vi "TwReadRawData.vi"(3 "error in (no error)":errorcluster, 4 "buffer":u8[](array[numeric]), 5 "filename":string, 6 "bufferSize in":i32, 7 "writeIndex":i32, 8 "bufIndex":i32, 9 "channel":i32) -> (0 "buffer out":u8[](array[numeric]), 1 "bufferSize out":i32, 2 "error out":errorcluster)   [LabVIEW 2009]
uses:
  TwH5Dll.dll
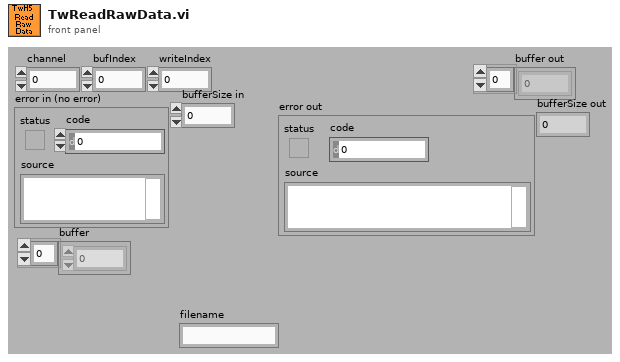
[diagram p1: front panel]
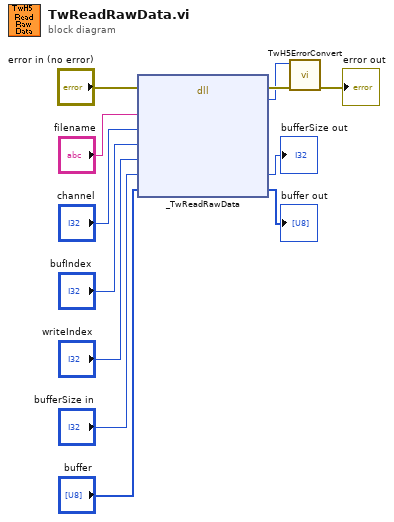
[diagram p0: block diagram]
diagram:
  n1 = dll-call lib="C:/src/85_TofDaq_current/DllWrappers/LabView/TwH5Dll/TwH5Dll.dll" fn="_TwReadRawData"(error in="error in (no error)", "filename"="filename", "channel"="channel", "bufIndex"="bufIndex", "writeIndex"="writeIndex", "bufferSize"="bufferSize in", "buffer"="buffer") -> (error out=w11:errorcluster, "TwRetVal"=w10:i32, "bufferSize"=→"bufferSize out":i32, "buffer"=→"buffer out":u8[])  [unwired: 6 in, 1 out]
  n2 = call "TwH5ErrorConvert.vi"("error in (no error)"=w11, "error code"=w10) -> ("error out"=→"error out":errorcluster)  [unwired: 9 out]
